vi "运行时菜单.vi"   [LabVIEW 2018]
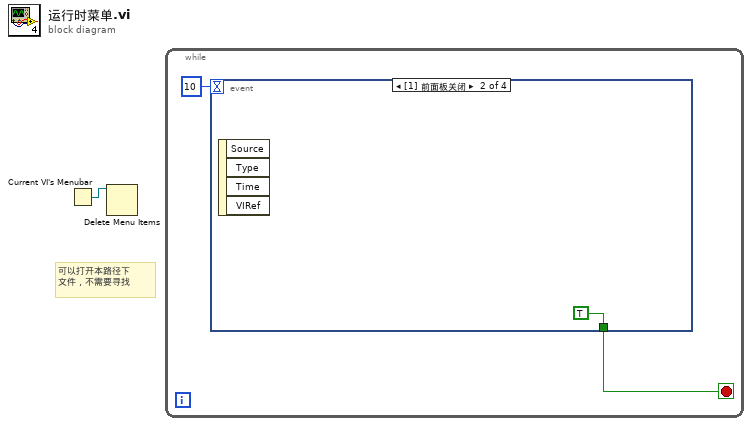
[diagram p0: block diagram]
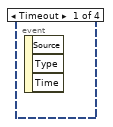
[diagram p2: hidden frame]
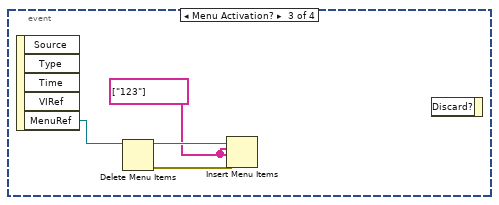
[diagram p3: hidden frame]
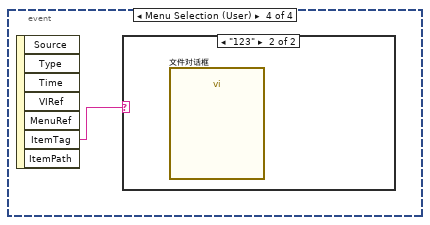
[diagram p4: hidden frame]
diagram:
  # "可以打开本路径下\n文件，不需要寻找"
  n1 = Current VI's Menubar() -> (w1:refnum<k9>)
  n2 = Delete Menu Items(9:w1) -> ()  [unwired: 3 in, 2 out]
  n3 = while {
    stop <- w2 stop-if-true
    n4 = event shown="[1] 前面板关闭" {
      selector: _ -> [_ _ _ _]
      dyn-events: _ -> [_ _ _ _]
      timeout: 10 -> [_ _ _ _]
      tunnel: [_ TRUE ("停止") _ _] -> w2
      event Timeout {
        n5 = event-data() -> ()  [unwired: 1 in, 3 out]
      }
      event Panel Close {
        n6 = event-data() -> ()  [unwired: 1 in, 4 out]
      }
      event Menu Activation? {
        w6 = string[] ["123"] ("项标识符")
        n7 = event-data() -> ("MenuRef"=w8:refnum<k9>)  [unwired: 1 in, 4 out]
        n8 = Delete Menu Items(9:w8) -> (0:w5:errorcluster, 3:w7:refnum<k9>)  [unwired: 3 in]
        n9 = Insert Menu Items(6:w5, 7:w6, 8:w6, 9:w7) -> ()  [unwired: 2 in, 3 out]
        n10 = event-data() -> ()  [unwired: 2 in, 1 out]
      }
      event Menu Selection (User) {
        n11 = event-data() -> ("ItemTag"=w9:string)  [unwired: 1 in, 6 out]
        n12 = case shown="\"123\"" w9 {
          frame "假", Default {
          }
          frame "123" {
            n13 = call "文件对话框"() -> ()  [unwired: 12 in, 4 out]
          }
        }
      }
    }
  }
